vi "HMI.vi"(8 "error in (no error)":errorcluster caption="entrée d'erreur (pas d'erreur)", 11 "Class Popup Operator_Validation (Default) en entrée":refnum<class "Class Popup Operator_Information.lvclass">) -> (0 "error out":errorcluster caption="sortie d'erreur", 1 "Input":string, 2 "Operator_Selection":bool, 3 "Class Popup Operator_Validation (Default) en sortie":refnum<class "Class Popup Operator_Information.lvclass">)   [LabVIEW 2020, in "Library Instrument & Equipement.lvlib" / "Library Popup.lvlib" / "Class Popup Operator_Information.lvclass"]
uses:
  Class Popup Operator_Information.lvclass
  C:/Users/ngarcin/OneDrive - Altyor/Standard TB/Class/Popup/Class Popup (Main)/Class Popup (Main).lvclass
  C:/Users/ngarcin/OneDrive - Altyor/Standard TB/Class/Popup/Class Popup Operator_Validation/Class Popup Operator_Validation (Default)/Class Popup Operator_Validation (Virtual).lvclass
  JSON API/JSON Value/Set from JSON string.vi
  JSON API/JSON Value/JSON Value.lvclass
  Class Popup Operator_Validation (Default)/Class Popup Operator_Validation (Virtual).lvclass
  Class Popup Operator_Information.lvclass/Class Popup Operator_Information.ctl
  JSON API/Variant JSON/Variant JSON.lvlib
  JSON API/Get Polymorphic/JSON GetSet.lvlib
panel:
  out "Text":string
  out "Image":picture
  in  "Bouton NOK":bool caption="Default"
  in  "Bouton OK":bool caption="Validated"
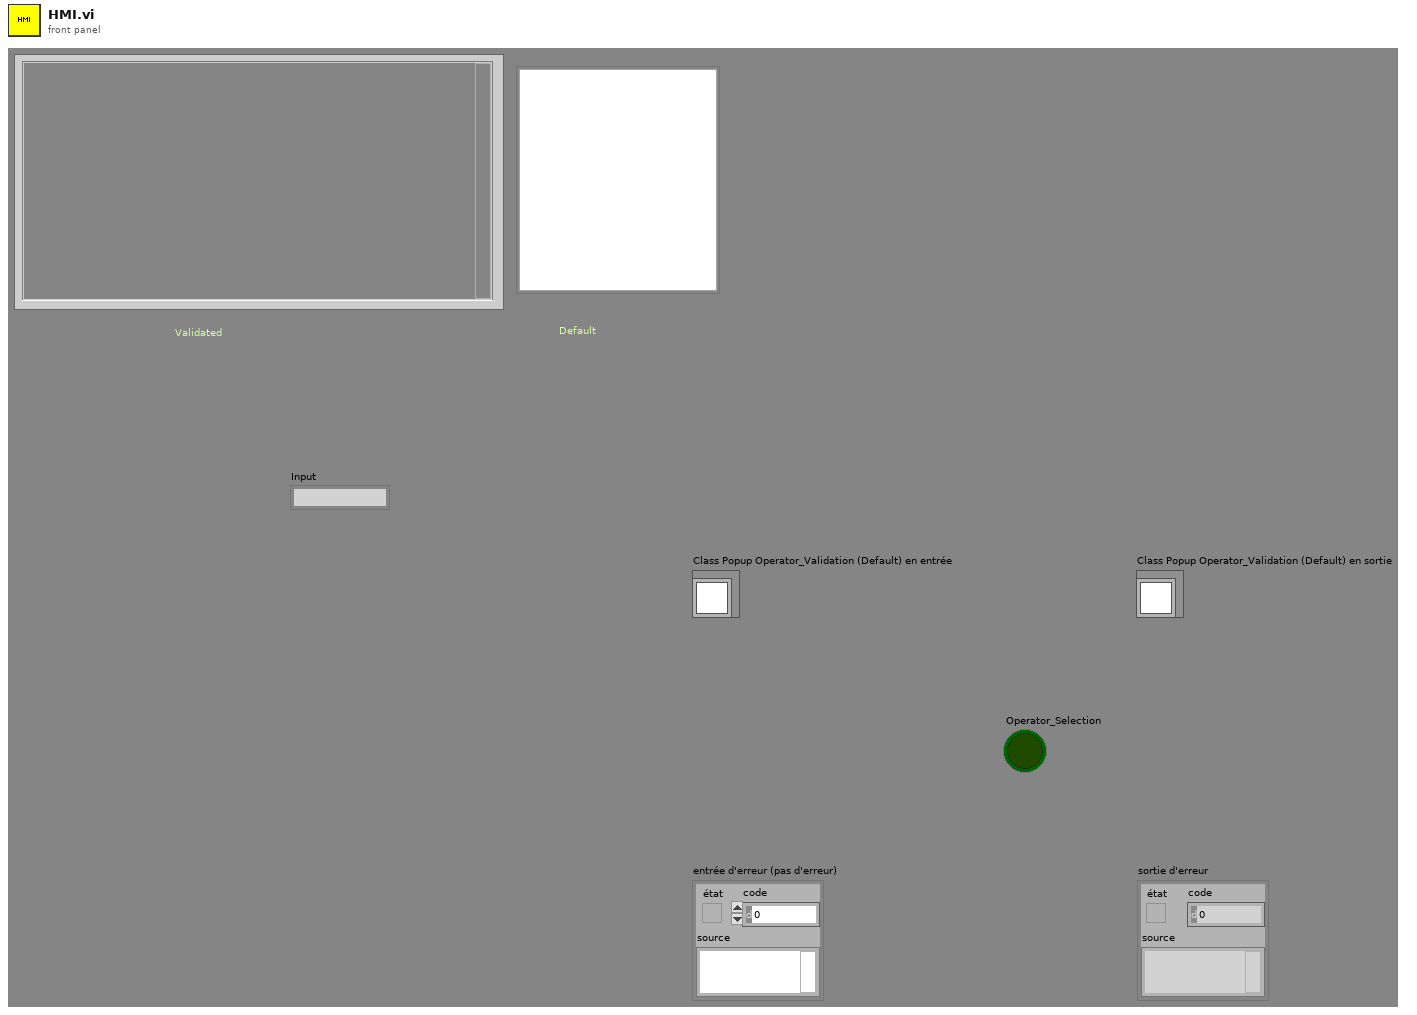
[diagram p1: front panel]
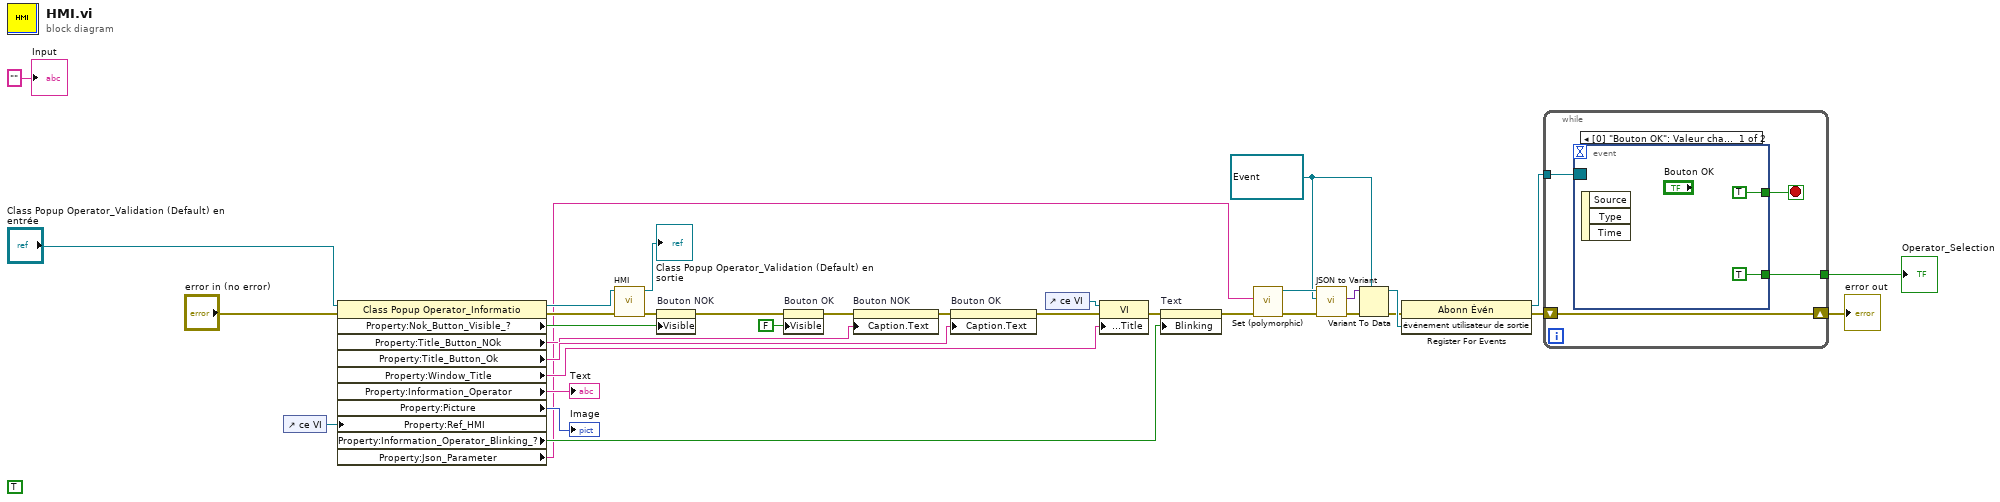
[diagram p0: block diagram]
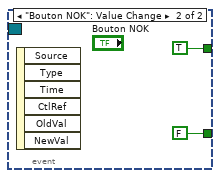
[diagram p2: hidden frame]
diagram:
  (unwired) TRUE ("données d'événement")
  w7 = refnum<user-event> refnum ("événement utilisateur de sortie")
  n1 = control-ref of="ce VI"() -> (w19:refnum<vi>)
  n2 = property class="Class Popup Operator_Informatio"(reference="Class Popup Operator_Validation (Default) en entrée", error in="error in (no error)", "Property:Ref_HMI"=w19) -> (reference out=w24:refnum<class "Class Popup Operator_Information.lvclass">, error out=w26:errorcluster, "Property:Nok_Button_Visible_?"=w35:bool, "Property:Title_Button_NOk"=w32:string, "Property:Title_Button_Ok"=w33:string, "Property:Window_Title"=w30:string, "Property:Information_Operator"=→"Text":string, "Property:Picture"=→"Image":picture, "Property:Information_Operator_Blinking_?"=w22:bool, "Property:Json_Parameter"=w6:string)
  n3 = call-parent "HMI.vi"("error in (no error)"=w26, "Class Popup Operator_Validation (Default) en entrée"=w24) -> ("error out"=w25:errorcluster, "Class Popup Operator_Validation (Default) en sortie"=→"Class Popup Operator_Validation (Default) en sortie":refnum<class "Class Popup Operator_Information.lvclass">)  [unwired: 6 in, 2 out]
  n4 = property on="Bouton NOK" class="Bool"(error in=w25, "Visible"=w35) -> (error out=w18:errorcluster)  [unwired: 1 in, 1 out]
  n5 = property on="Bouton OK" class="Bool"(error in=w18, "Visible"=FALSE) -> (error out=w17:errorcluster)  [unwired: 1 in, 1 out]
  n6 = property on="Bouton NOK" class="Bool"(error in=w17, "Caption.Text"=w32) -> (error out=w16:errorcluster)  [unwired: 1 in, 1 out]
  n7 = property on="Bouton OK" class="Bool"(error in=w16, "Caption.Text"=w33) -> (error out=w14:errorcluster)  [unwired: 1 in, 1 out]
  n8 = control-ref of="ce VI"() -> (w15:refnum<vi>)
  n9 = property class="VI"(reference=w15, error in=w14, "Front Panel.Title"=w30) -> (error out=w13:errorcluster)  [unwired: 1 out]
  n10 = property on="Text" class="Ch"(error in=w13, "Blinking"=w22) -> (error out=w4:errorcluster)  [unwired: 1 in, 1 out]
  n11 = call-poly "Set (polymorphic).vi"("error in (no error)"=w4, "JSON stream"=w6) -> ("error out"=w9:errorcluster, "JSON Value out"=w11:refnum<class "JSON Value.lvclass">)  [unwired: 7 in, 1 out]
  n12 = call "JSON to Variant.vi"("error in (no error)"=w9, "Variant (Data Type)"=w7, "JSON Value"=w11) -> ("error out"=w10:errorcluster, "Variant out"=w8:variant)  [unwired: 7 in]
  n13 = Variant To Data(error in=w10, type=w7, Variant=w8) -> (data=w5:refnum<user-event>, error out=w3:errorcluster)
  n14 = register-events(error in=w3, w5) -> (reference out=w2:refnum<event-registration>, error out=w1:errorcluster)  [unwired: 1 in]
  n15 = while {
    tunnel: [w37] -> w31
    shift-right: [w38] -> w27
    shift-left: w1 -> [w38]
    tunnel: w2 -> [w36]
    stop <- w39 stop-if-true
    n16 = event shown="[0] \"Bouton OK\": Valeur changée;  <événement utilisateur de sortie>: Événement utilisateur" {
      selector: w36 -> [_ _]
      dyn-events: _ -> [_ _]
      timeout: _ -> [_ _]
      tunnel: [TRUE ("Valeur (Signalisation)") TRUE ("Valeur (Signalisation)")] -> w39
      tunnel: [TRUE ("Operator_Selection") FALSE ("Operator_Selection")] -> w37
      event "Bouton OK": Value Change; User Event {
        n17 = event-data() -> ()  [unwired: 1 in, 3 out]
      }
      event "Bouton NOK": Value Change {
        n18 = event-data() -> ()  [unwired: 1 in, 6 out]
      }
    }
  }
  "error out" <- w27
  "Operator_Selection" <- w31
  "Input" <- "" ("Input")
